vi "Find Line Indent.vi"(0 "Functions in":T1[](array[typedef]), 1 "Indent Identifier":string="//", 11 "error in (no error)":errorcluster) -> (4 "Functions":T1[](array[typedef]), 15 "error out":errorcluster)   [LabVIEW 2016]
uses:
  Line Details.ctl
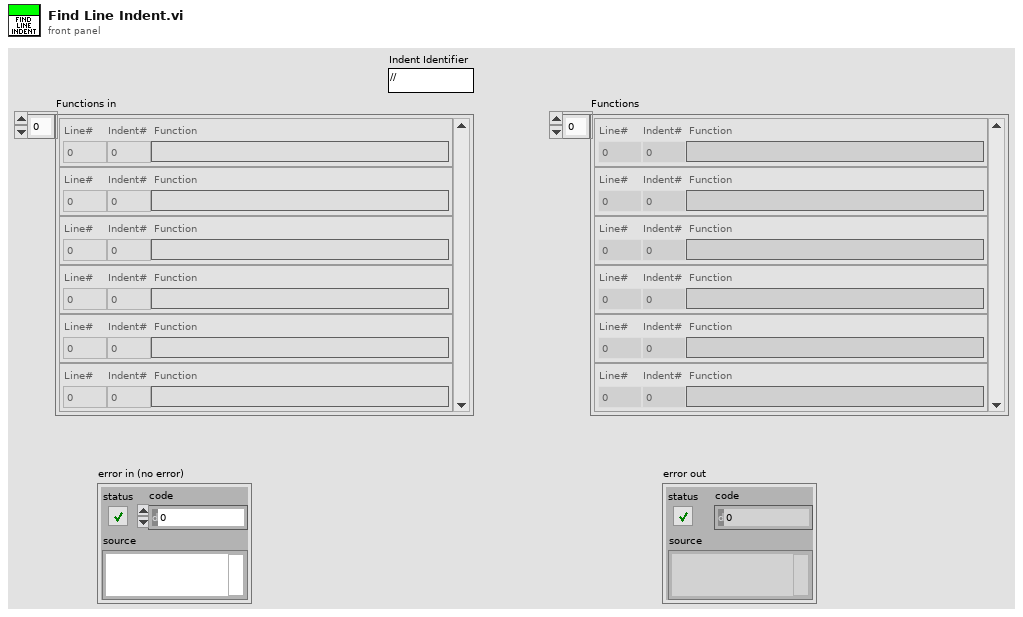
[diagram p1: front panel]
types:
  T1 = typedef "Line Details.ctl" = cluster{"Line#":i64, "Indent#":i64, "Function":string}
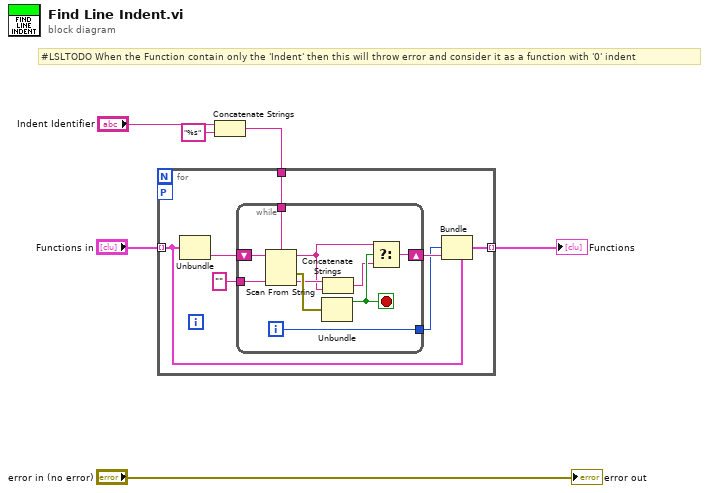
[diagram p0: block diagram]
diagram:
  # "#LSLTODO When the Function contain only the 'Indent' then this will throw error and consider it as a function with '0' indent"
  n1 = Concatenate Strings("Indent Identifier", "%s" ("string")) -> (w4:string)
  n2 = for {
    tunnel: "Functions in" -> [w9] mode=indexing
    tunnel: w4 -> [w13]
    tunnel: [w12] -> w1 mode=indexing
    workers-P: _ -> [_]
    n3 = Unbundle(w9) -> ("Function"=w10:string)  [unwired: 2 out]
    n4 = while {
      tunnel: w13 -> [w23]
      tunnel: [w21] -> w7
      tunnel: "" -> [w20]
      shift-right: [w16] -> w8
      shift-left: w10 -> [w19]
      i -> [w21]
      stop <- w18 stop-if-true
      n5 = Scan From String(format string=w23, input string=w19, default 1=w20) -> (remaining string=w14:string, error out=w22:errorcluster, output 1=w17:string)  [unwired: 2 in, 1 out]
      n6 = Unbundle(w22) -> ("status"=w18:bool)  [unwired: 2 out]
      n7 = Concatenate Strings(w17, w14) -> (w15:string)
      n8 = Select(t=w14, s=w18, f=w15) -> (s? t:f=w16:string)
    }
    n9 = Bundle(cluster=w9, "Indent#"=w7, "Function"=w8) -> (w12:T1)  [unwired: 1 in]
  }
  "Functions" <- w1
  "error out" <- "error in (no error)"
